vi "FFID_C_Profile.vi"(4 "Point Increment In":i32, 5 "Loop i":i32, 6 "Arguments":string[](array[string]), 7 "Simulate/Run":T1) -> (0 "Point Increment Out":i32, 2 "Error String":string, 3 "Continue":bool)   [LabVIEW 2015]
uses:
  Controls/User_Specific_mode.ctl
  Controls/Inst_type.ctl
  Globals/Meas_global.vi
  Globals/Trav_pos_global.vi
panel:
  out "Threshold":dbl
  out "Cut off %":dbl
  out "New Crossection?":bool
  out "Max value and position":dbl[](array[numeric])
  out "Indexes":i32[](array[numeric])
  out "Crossection Name":string
  out "Current Concentrations":dbl[](array[numeric])
  # "Cmax\n\n\nX  at Cmax\n\nY at Cmax\n\nZ at Cmax\n\n\nXmin\n\nXmax\n\n\nYmin\n\nYmax\n\n\nZmin\n\nZmax"
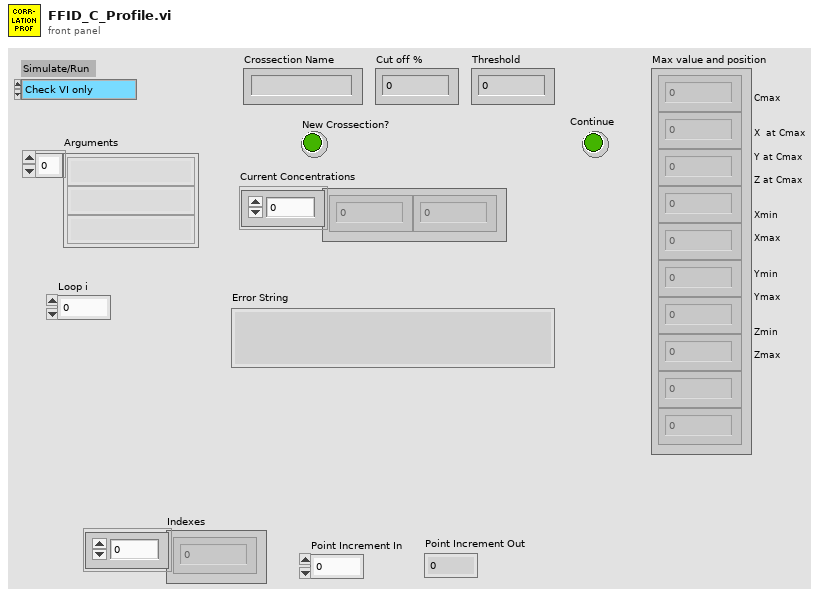
[diagram p1: front panel]
types:
  T1 = typedef "User_Specific_mode.ctl" = enum16{"Check VI only", "Run VI"}
  T2 = typedef "Traverse_cluster.ctl" = cluster{"Start X":sgl, "Start Y":sgl, "Start Z":sgl, "End X":sgl, "End Y":sgl, "End Z":sgl, "No. of pts.":i32, "Spacing":T3, "Filename":path, "Tunnel Speed":dbl, "Averaging time (min)":dbl, "Extra Commands":string, "Carrier_1 Q (l/min)":dbl, "Carrier_2 Q (l/min)":dbl, "Trace Gas Concentration (%)":dbl, "Specific Arguments":string, "Comments":string, "Row No":i32, "Row Type Selector":T4, "Completion time":string, "Row Duration (mins)":dbl, "No. of Valid pts.":i32, "Meas Setup File":string}
  T3 = typedef "Spacing.ctl" = enum16{"Linear", "Log", "Gauss", "Specified", "N/A"}
  T4 = typedef "Multi_run_mode.ctl" = enum16{"Move Traverse Only", "Set Tunnel Speed Only", "Set Source Only", "Set Measurement Conditions", "Single Measurement", "Vertical Profile", "Lateral Profile", "Longitudinal Profile", "Explore Volume", "Multi-Axis Profile", "Auto Calibrate", "Meas Fast FID Bkgnd", "Check Beam Power", "Scanning Valve Measurement", "Run VI Named:", "Set ADAM Ch", "Wait (minutes)", "Send Message", "Synchronize With:", "Fall Back to this Row", "Turn Off Row Repeating", "Blank Row", "Traverse 3D Volume"}
  T5 = typedef "Analysis_info_cluster.ctl" = cluster{"Colour":u32, "Inst type":T6, "Inst name":string, "Symbol":string, "Code name":string, "Extra Info":string, "Inst Array":T7, "Extra Titles":string[], "Extra Values":string[], "U":dbl, "u^2":dbl, "u^3":dbl, "u^4":dbl, "Skew_u":dbl, "Kurt_u":dbl, "Sd Error in Mean":dbl, "% u'/U":dbl, "X":dbl, "Y":dbl, "Z":dbl, "Timescale integral to 25%":dbl, "Sd Error in Variance":dbl, "Calib File":path, "Calib Constants":dbl[], "Output Position":bool, "Full Stats":bool, "Av Sampling Rate":dbl, "Av No of Samples":dbl, "Total Meas Time (s)":dbl, "ADAM Ch Name":string, "Max value":dbl, "Min value":dbl}
  T6 = typedef "Inst_type.ctl" = enum16{"Propeller anemometer", "Raw voltage", "Pressure Transducer", "Pitot-static tube", "Preston tube", "Hot wire", "Cross wire 1", "Cross wire 2", "Generic Linear", "Generic Polynomial", "Generic BackPoly", "Fast FID", "Thermocouple", "Cold wire", "Pulsed Wire", "LDA Vel", "LDA Tran time", "LDA Arr time", "Microphone"}
  T7 = typedef "Instrument_Array.ctl" = enum16{"PWA", "LDA", "Analogue"}
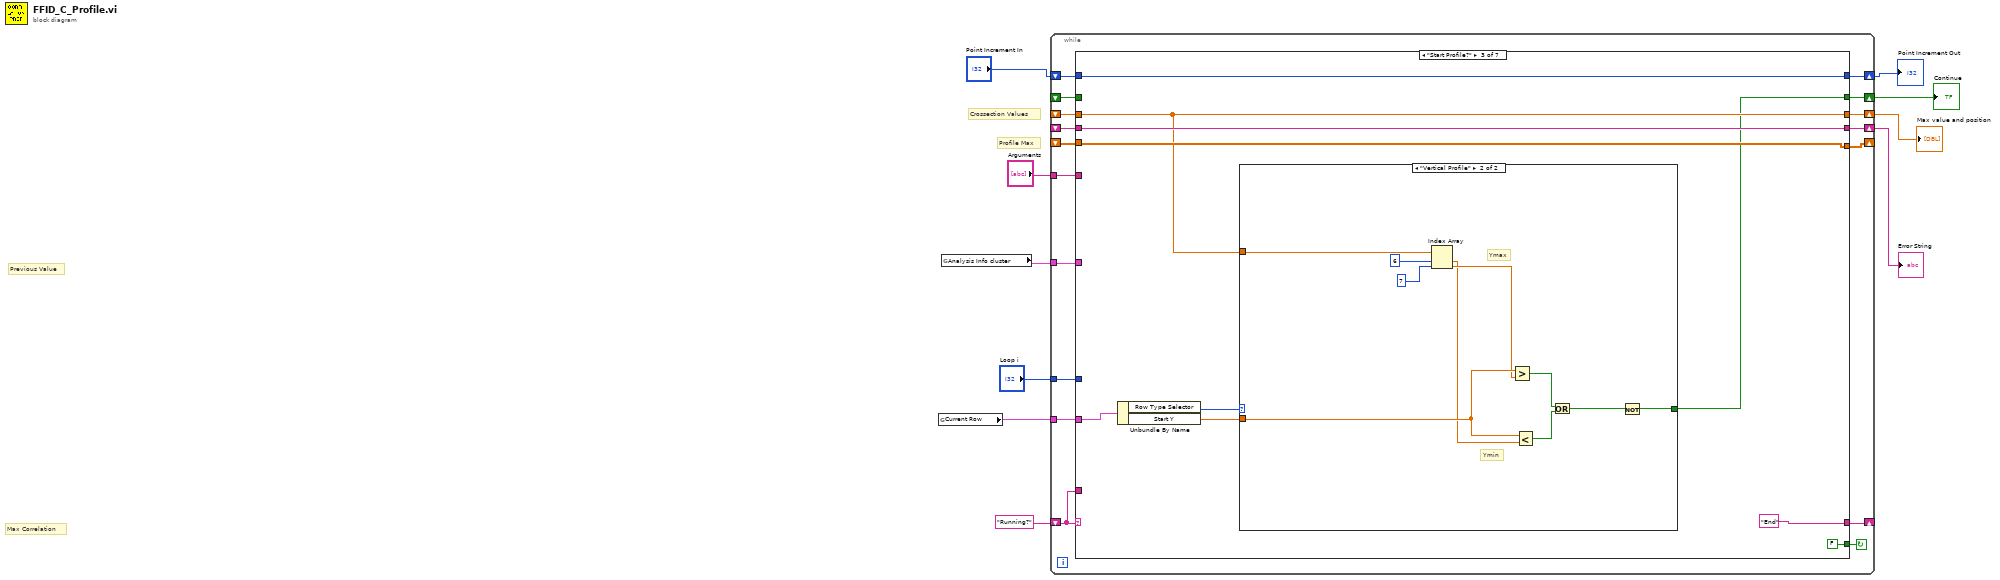
[diagram p0: block diagram]
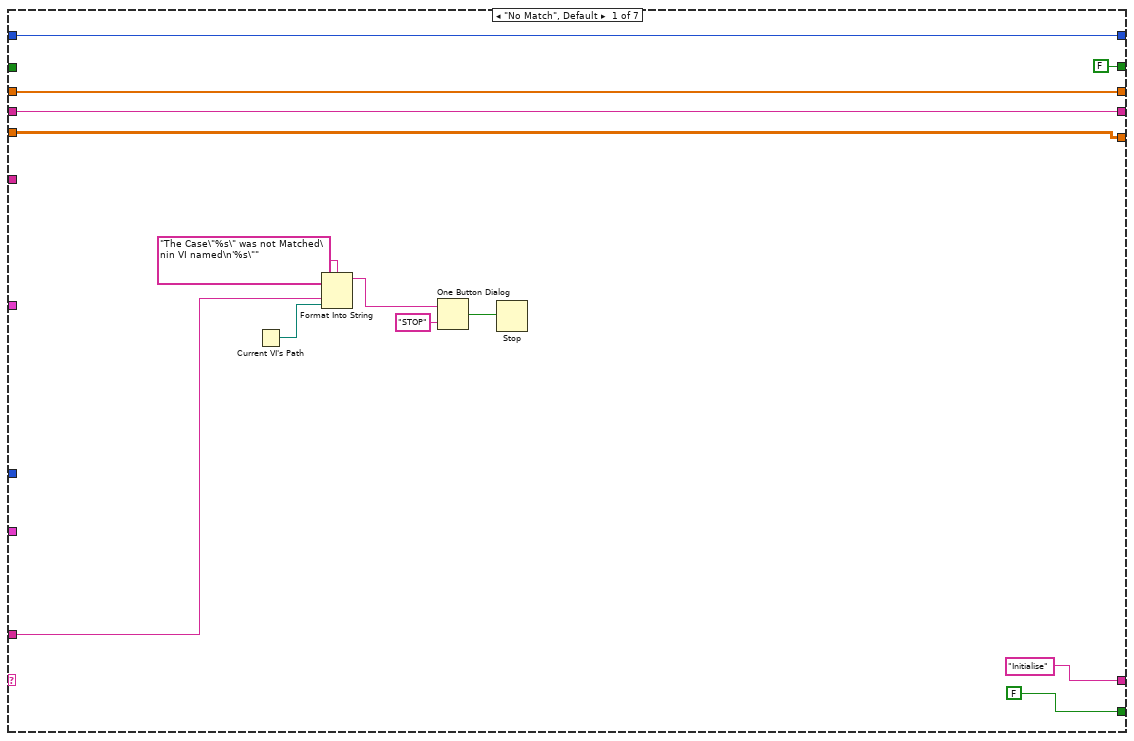
[diagram p2: hidden frame]
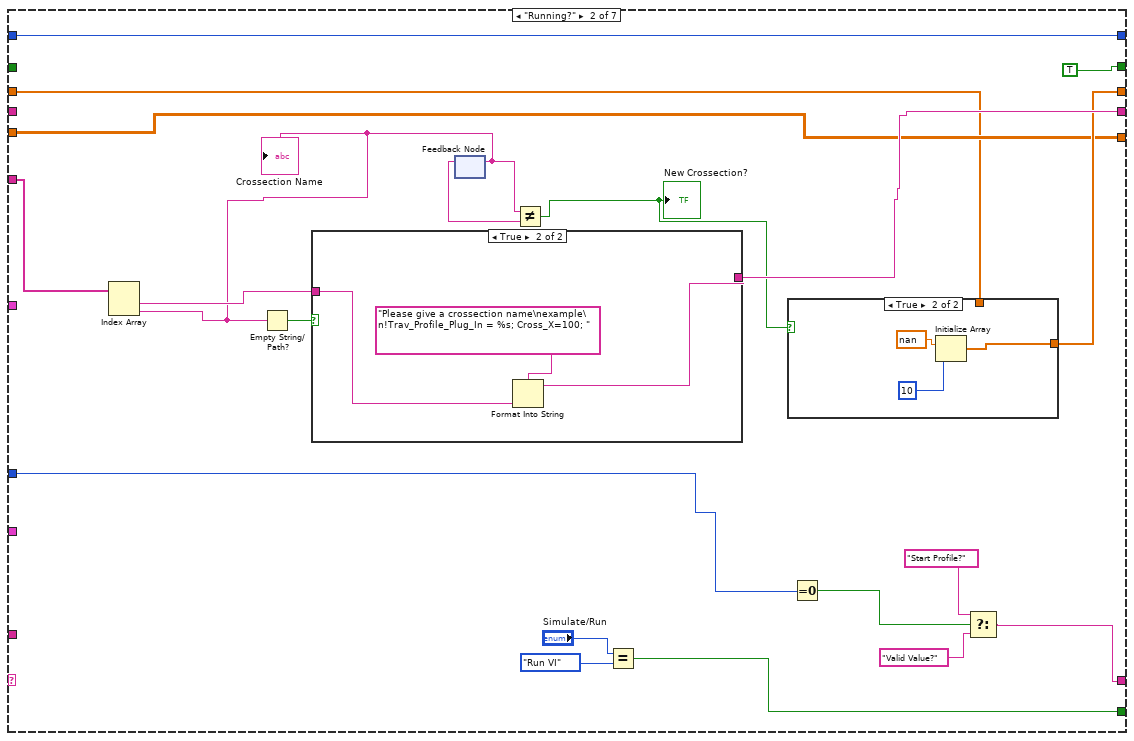
[diagram p3: hidden frame]
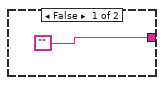
[diagram p5: hidden frame]
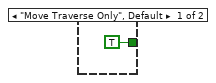
[diagram p6: hidden frame]
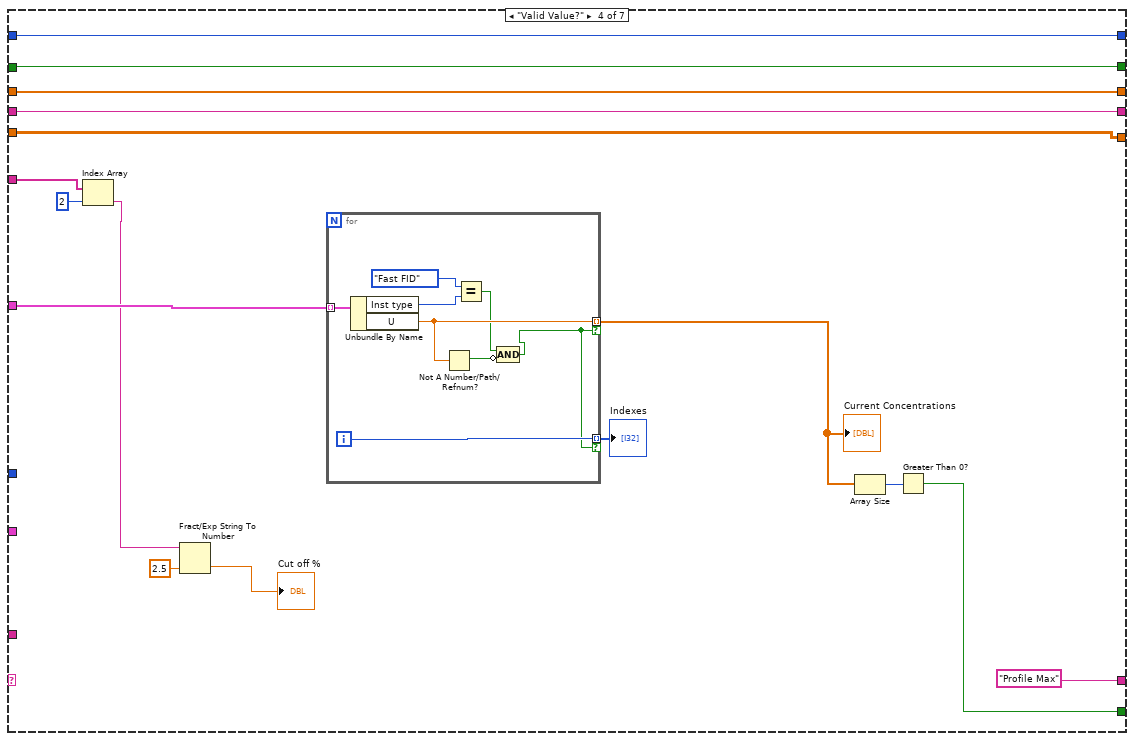
[diagram p7: hidden frame]
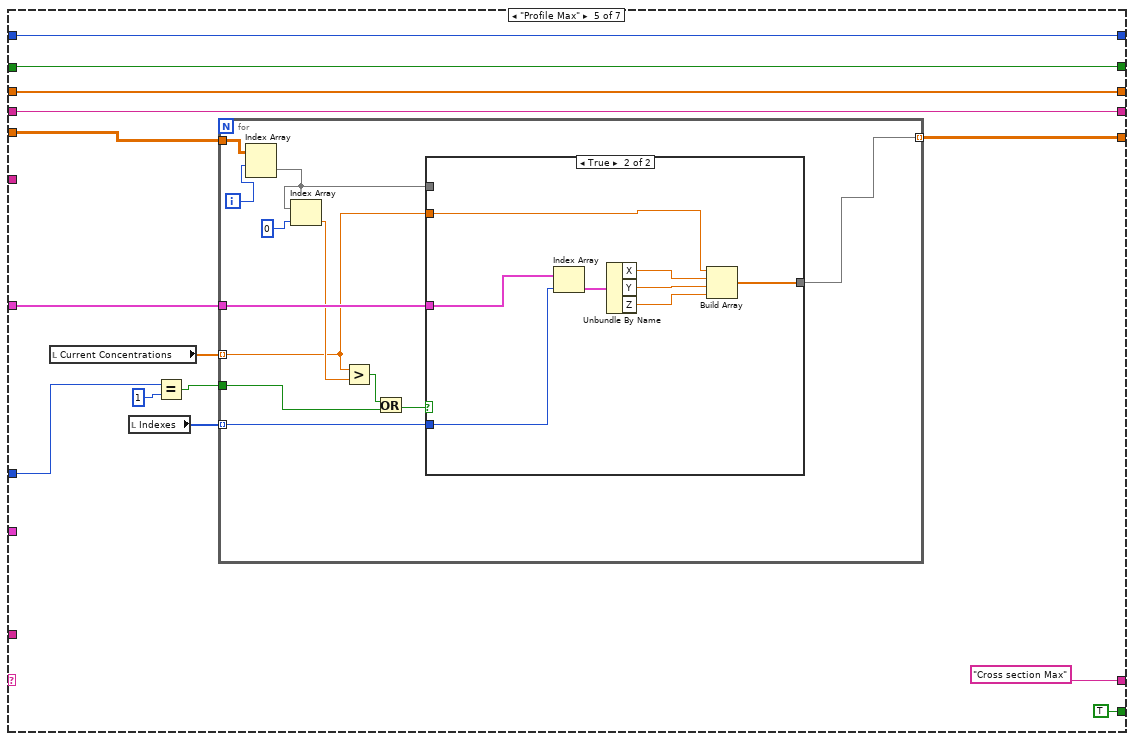
[diagram p8: hidden frame]
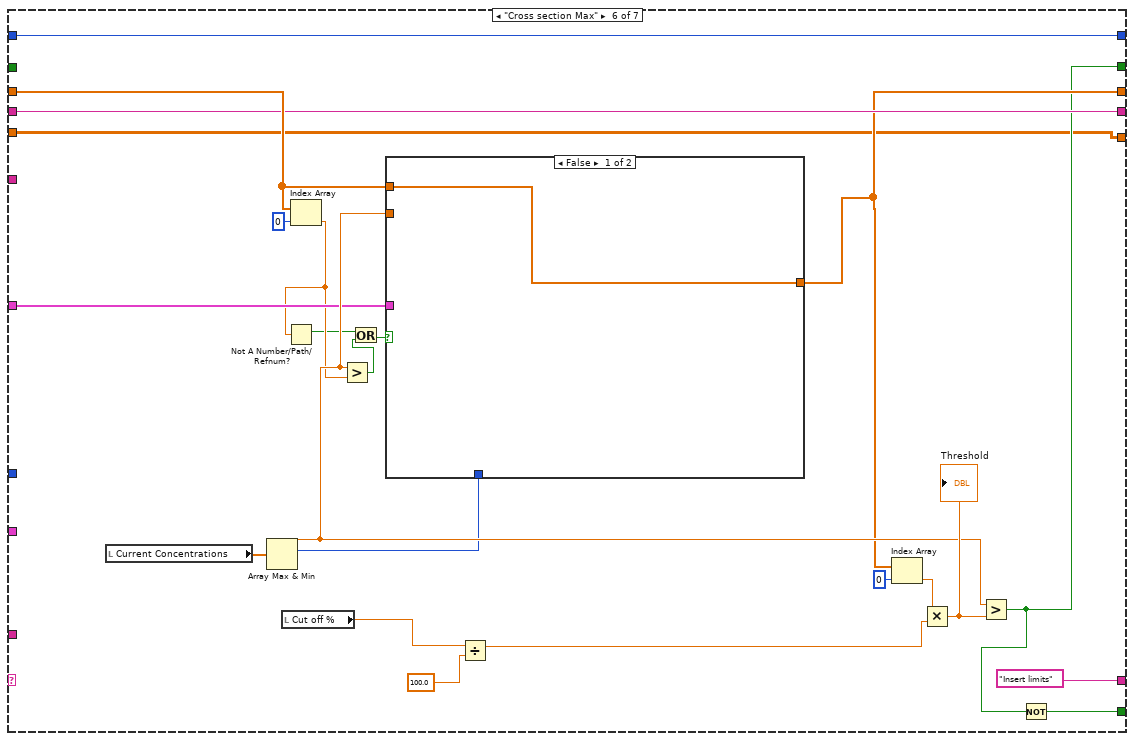
[diagram p10: hidden frame]
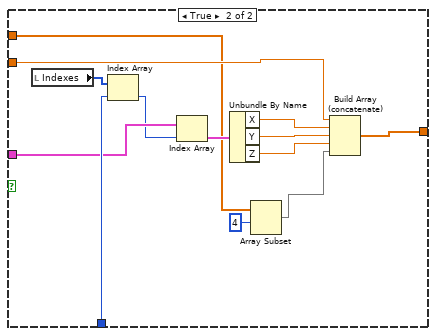
[diagram p11: hidden frame]
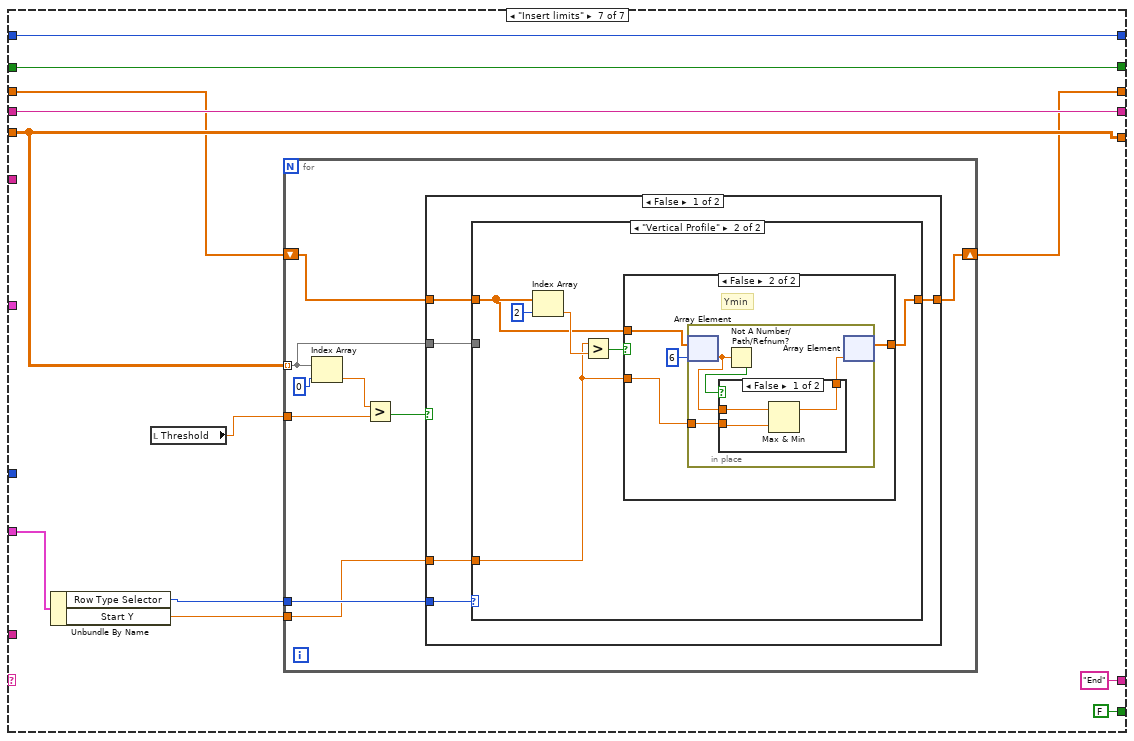
[diagram p12: hidden frame]
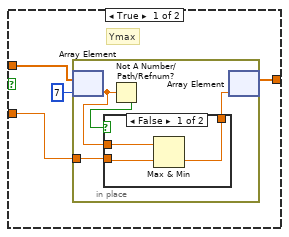
[diagram p14: hidden frame]
diagram:
  # "Profile Max"
  # "Crossection Values"
  # "Previous Value"
  # "Max Correlation"
  n1 = global read "Trav_pos_global.vi" "Current Row"() -> (w1:T2)
  n2 = global read "Meas_global.vi" "Analysis Info cluster"() -> (w3:T5[])
  n3 = while {
    shift-left: "Running?" -> [w25]
    shift-right: [w26] -> _
    shift-right: [w23] -> w8
    shift-left: "Point Increment In" -> [w24]
    shift-right: [w22] -> w7
    shift-left: _ -> [w21]
    shift-right: [w20] -> w2
    shift-left: _ -> [w19]
    tunnel: "Arguments" -> [w18]
    shift-right: [w17] -> w5
    shift-left: _ -> [w16]
    tunnel: "Loop i" -> [w15]
    tunnel: w3 -> [w14]
    shift-right: [w12] -> _
    shift-left: _ -> [w13]
    tunnel: w1 -> [w11]
    stop <- w27 continue-if-true
    n4 = case shown="\"Start Profile?\"" w25 {
      tunnel: [FALSE w56 FALSE w99 TRUE w150 FALSE] -> w27
      tunnel: ["Initialise" w42 "End" "Profile Max" "Cross section Max" "Insert limits" "End" ("t")] -> w26
      tunnel: w25 -> [w35 _ _ _ _ _ _]
      tunnel: w24 -> [w32 w58 w77 w103 w125 w170 w197]
      tunnel: [w32 w58 w77 w103 w125 w170 w197] -> w23
      tunnel: [FALSE TRUE w70 w104 w118 w151 w196] -> w22
      tunnel: w21 -> [_ _ _ w104 w118 _ w196]
      tunnel: [w30 w49 w72 w102 w119 w159 w191] -> w20
      tunnel: w19 -> [w30 w47 w72 w102 w119 w168 w192]
      tunnel: w18 -> [_ w55 _ w94 _ _ _]
      tunnel: [w29 w53 w76 w98 w124 w163 w195] -> w17
      tunnel: w16 -> [w29 _ w76 w98 w124 w163 w195]
      tunnel: w15 -> [_ w43 _ _ w117 _ _]
      tunnel: w14 -> [_ _ _ w96 w123 w161 _]
      tunnel: w13 -> [w28 w48 w75 w91 w120 w149 w194]
      tunnel: [w28 w48 w75 w91 w114 w149 w194] -> w12
      tunnel: w11 -> [_ _ w74 _ _ _ w187]
      frame "No Match", Default {
        n5 = Current VI's Path() -> (path=w34:path)
        n6 = Format Into String(format string="The Case\"%s\" was not Matched\nin VI named\n'%s\"" ("Format String"), w35, w34) -> (resulting string=w38:string)  [unwired: 2 in, 1 out]
        n7 = One Button Dialog(message=w38, button name ("OK")="STOP") -> (true=w36:bool)
        n8 = Stop(stop? (T)=w36) -> ()
      }
      frame "Running?" {
        n9 = Index Array(array=w55) -> (element #1=w51:string, element #2=w41:string)  [unwired: 2 in]
        "Crossection Name" <- w41
        n10 = Empty String/Path?(string/path=w41) -> (empty?=w54:bool)
        n11 = case shown="True" w54 {
          tunnel: ["" w66] -> w53
          tunnel: w51 -> [_ w68]
          frame False {
          }
          frame True {
            n12 = Format Into String(format string="Please give a crossection name\nexample\n!Trav_Profile_Plug_In = %s; Cross_X=100; ", w68) -> (resulting string=w66:string)  [unwired: 2 in, 1 out]
          }
        }
        n13 = feedback #1() -> (w52:string)  [unwired: 1 in]
        n14 = feedback-in #1(w41) -> ()
        n15 = Not Equal?(x=w41, y=w52) -> (x != y?=w50:bool)
        "New Crossection?" <- w50
        n16 = Equal?(x="Simulate/Run", y=User_Specific_mode."Run VI" ("Simulate/Run")) -> (x = y?=w56:bool)
        n17 = case shown="True" w50 {
          tunnel: [w61 w62] -> w49
          tunnel: w47 -> [w61 _]
          frame False {
          }
          frame True {
            n18 = Initialize Array(nan, 10 ("dimension size")) -> (w62:dbl[])
          }
        }
        n19 = Equal To 0?(x=w43) -> (x = 0?=w45:bool)
        n20 = Select(t="Start Profile?", s=w45, f="Valid Value?") -> (s? t:f=w42:string)
      }
      frame "Start Profile?" {
        n21 = Unbundle By Name(w74) -> ("Row Type Selector"=w73:T4, "Start Y"=w71:sgl)
        n22 = case shown="\"Vertical Profile\"" w73 {
          tunnel: w72 -> [_ w89]
          tunnel: w71 -> [_ w87]
          tunnel: [TRUE w88] -> w70
          frame "Move Traverse Only", Default {
          }
          frame "Vertical Profile" {
            # "Ymax"
            # "Ymin"
            n23 = Index Array(array=w89, index #1=6 ("index"), index #2=7 ("index")) -> (element #1=w83:dbl, element #2=w84:dbl)
            n24 = Greater?(x=w87, y=w84) -> (0:w81:bool)
            n25 = Less?(x=w87, y=w83) -> (x < y?=w82:bool)
            n26 = Or(x=w81, y=w82) -> (x .or. y?=w80:bool)
            n27 = Not(x=w80) -> (.not. x?=w88:bool)
          }
        }
      }
      frame "Valid Value?" {
        n28 = Index Array(array=w94, index=2) -> (element=w90:string)
        n29 = Fract/Exp String To Number(string=w90, default (0 dbl)=2.5 ("default (0 DBL)")) -> (number=→"Cut off %":dbl)  [unwired: 2 in, 1 out]
        n30 = for {
          tunnel: w96 -> [w113] mode=indexing
          tunnel: [w110] -> w101 mode=indexing if=w106
          tunnel: [w107] -> w97 mode=indexing if=w106
          i -> [w107]
          n31 = Unbundle By Name(w113) -> ("Inst type"=w112:T6, "U"=w110:dbl)
          n32 = Not A Number/Path/Refnum?(number/path/refnum=w110) -> (NaN/Path/Refnum?=w109:bool)
          n33 = Equal?(x=Inst_type."Fast FID" ("Inst type"), y=w112) -> (x = y?=w108:bool)
          n34 = Compound Arithmetic op=AND(w108, invert w109) -> (w106:bool)
        }
        "Current Concentrations" <- w101
        "Indexes" <- w97
        n35 = Array Size(array=w101) -> (size(s)=w100:i32)
        n36 = Greater Than 0?(x=w100) -> (x > 0?=w99:bool)
      }
      frame "Profile Max" {
        n37 = local read "Current Concentrations"() -> (w121:dbl[])
        n38 = local read "Indexes"() -> (w122:i32[])
        n39 = Equal?(x=w117, y=1) -> (x = y?=w115:bool)
        n40 = for {
          tunnel: w123 -> [w139]
          tunnel: w122 -> [w138] mode=indexing
          tunnel: w121 -> [w135] mode=indexing
          tunnel: w115 -> [w133]
          tunnel: w120 -> [w130]
          tunnel: [w132] -> w114 mode=indexing
          i -> [w131]
          n41 = Index Array(array=w130, index (row)=w131) -> (element=w129:dbl[])  [unwired: 1 in]
          n42 = Index Array(array=w129, index=0) -> (element=w137:dbl)
          n43 = Greater?(x=w135, y=w137) -> (0:w134:bool)
          n44 = Or(x=w134, y=w133) -> (x .or. y?=w136:bool)
          n45 = case shown="True" w136 {
            tunnel: w139 -> [_ w148]
            tunnel: w135 -> [_ w143]
            tunnel: [w140 w142] -> w132
            tunnel: w129 -> [w140 _]
            tunnel: w138 -> [_ w141]
            frame False {
            }
            frame True {
              n46 = Index Array(array=w148, index=w141) -> (element=w147:T5)
              n47 = Unbundle By Name(w147) -> ("X"=w144:dbl, "Y"=w145:dbl, "Z"=w146:dbl)
              n48 = Build Array(w143, w144, w145, w146) -> (w142:dbl[])
            }
          }
        }
      }
      frame "Cross section Max" {
        n49 = local read "Current Concentrations"() -> (w169:dbl[])
        n50 = Array Max & Min(array=w169) -> (max value=w164:dbl, max index (indices)=w162:i32)  [unwired: 2 out]
        n51 = local read "Cut off %"() -> (w157:dbl)
        n52 = Index Array(array=w168, index=0) -> (element=w155:dbl)
        n53 = Not A Number/Path/Refnum?(number/path/refnum=w155) -> (NaN/Path/Refnum?=w153:bool)
        n54 = Greater?(x=w164, y=w155) -> (0:w154:bool)
        n55 = Or(x=w153, y=w154) -> (x .or. y?=w152:bool)
        n56 = case shown="False" w152 {
          tunnel: w162 -> [_ w184]
          tunnel: w161 -> [_ w183]
          tunnel: w164 -> [_ w177]
          tunnel: [w172 w176] -> w159
          tunnel: w168 -> [w172 w175]
          frame False {
          }
          frame True {
            n57 = local read "Indexes"() -> (w185:i32[])
            n58 = Index Array(array=w185, index=w184) -> (element=w182:i32)
            n59 = Index Array(array=w183, index=w182) -> (element=w181:T5)
            n60 = Unbundle By Name(w181) -> ("X"=w178:dbl, "Y"=w179:dbl, "Z"=w180:dbl)
            n61 = Array Subset(array=w175, index=4) -> (w173:dbl[])  [unwired: 1 in]
            n62 = Build Array (concatenate)(w177, w178, w179, w180, w173) -> (w176:dbl[])
          }
        }
        n63 = Divide(x=w157, y=100.0) -> (x/y=w166:dbl)
        n64 = Index Array(array=w159, index=0) -> (element=w158:dbl)
        n65 = Multiply(x=w158, y=w166) -> (x*y=w165:dbl)
        "Threshold" <- w165
        n66 = Greater?(x=w164, y=w165) -> (0:w151:bool)
        n67 = Not(x=w151) -> (.not. x?=w150:bool)
      }
      frame "Insert limits" {
        n68 = Unbundle By Name(w187) -> ("Row Type Selector"=w188:T4, "Start Y"=w186:sgl)
        n69 = local read "Threshold"() -> (w193:dbl)
        n70 = for {
          tunnel: w194 -> [w201] mode=indexing
          tunnel: w193 -> [w204]
          tunnel: w188 -> [w202]
          shift-right: [w199] -> w191
          shift-left: w192 -> [w200]
          tunnel: w186 -> [w198]
          n71 = Index Array(array=w201, index=0) -> (element=w205:dbl)
          n72 = Greater?(x=w205, y=w204) -> (0:w203:bool)
          n73 = case shown="False" w203 {
            tunnel: w202 -> [w211 _]
            tunnel: w200 -> [w210 w243]
            tunnel: w201 -> [w209 _]
            tunnel: [w208 w243] -> w199
            tunnel: w198 -> [w207 _]
            frame False {
              n74 = case shown="\"Vertical Profile\"" w211 {
                tunnel: w210 -> [w212 w215]
                tunnel: w209 -> [_ _]
                tunnel: [w212 w214] -> w208
                tunnel: w207 -> [_ w213]
                frame "Move Traverse Only", Default {
                }
                frame "Vertical Profile" {
                  n75 = Index Array(array=w215, index=2) -> (element=w217:dbl)
                  n76 = Greater?(x=w213, y=w217) -> (0:w216:bool)
                  n77 = case shown="False" w216 {
                    tunnel: w215 -> [w222 w234]
                    tunnel: w213 -> [w220 w232]
                    tunnel: [w219 w231] -> w214
                    frame True {
                      # "Ymax"
                      n78 = in-place {
                        in-place-border: w220 -> [w224]
                        n79 = in-place-array #2(w222, 7) -> (w223:dbl)
                        n80 = Not A Number/Path/Refnum?(number/path/refnum=w223) -> (NaN/Path/Refnum?=w226:bool)
                        n81 = case shown="False" w226 {
                          tunnel: [w227 w230] -> w225
                          tunnel: w224 -> [w229 w230]
                          tunnel: w223 -> [w228 _]
                          frame False {
                            n82 = Max & Min(x=w228, y=w229) -> (min(x,y)=w227:dbl)  [unwired: 1 out]
                          }
                          frame True {
                          }
                        }
                        n83 = in-place-array #2(w225) -> (w219:dbl[])  [unwired: 1 out]
                      }
                    }
                    frame False {
                      # "Ymin"
                      n84 = in-place {
                        in-place-border: w232 -> [w236]
                        n85 = in-place-array #3(w234, 6) -> (w235:dbl)
                        n86 = Not A Number/Path/Refnum?(number/path/refnum=w235) -> (NaN/Path/Refnum?=w238:bool)
                        n87 = case shown="False" w238 {
                          tunnel: [w239 w242] -> w237
                          tunnel: w236 -> [w241 w242]
                          tunnel: w235 -> [w240 _]
                          frame False {
                            n88 = Max & Min(x=w240, y=w241) -> (max(x,y)=w239:dbl)  [unwired: 1 out]
                          }
                          frame True {
                          }
                        }
                        n89 = in-place-array #3(w237) -> (w231:dbl[])  [unwired: 1 out]
                      }
                    }
                  }
                }
              }
            }
            frame True {
            }
          }
        }
      }
    }
  }
  "Point Increment Out" <- w8
  "Continue" <- w7
  "Error String" <- w5
  "Max value and position" <- w2
